vi "Get Display String.vi"(11 "Str Starts With in":refnum<class "Str Starts With.lvclass">) -> (2 "Display String":string)   [LabVIEW 2018, in "Str Starts With.lvclass"]
uses:
  Str Starts With.lvclass
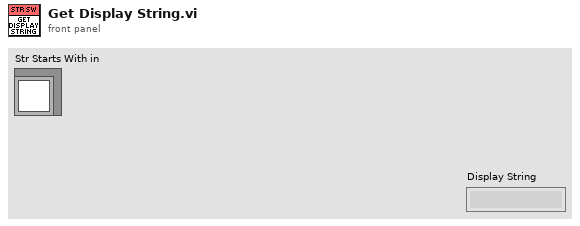
[diagram p1: front panel]
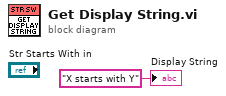
[diagram p0: block diagram]
diagram:
  "Display String" <- "X starts with Y" ("Display String")
